vi "Init and Generation Duration.vi"(8 "error in":errorcluster) -> (0 "Generated Error":errorcluster, 2 "Generation Duration [ms]":dbl, 3 "Init Duration [ms]":dbl)   [LabVIEW 2021]
doc: "Measure the duration of <b>Init Error Handler</b> function with 1000 error codes in XML as an input. The resulting duration is returned at <b>Init Duration [ms]</b> output. \nThe time of <b>Generate Error</b> function with no input to format is also measured and returned at <b>Generation Duration [ms]</b> output."
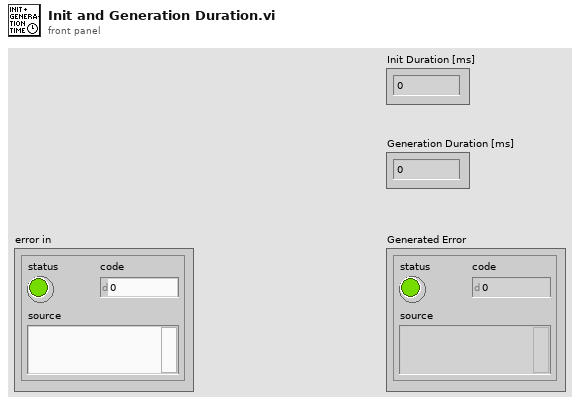
[diagram p1: front panel]
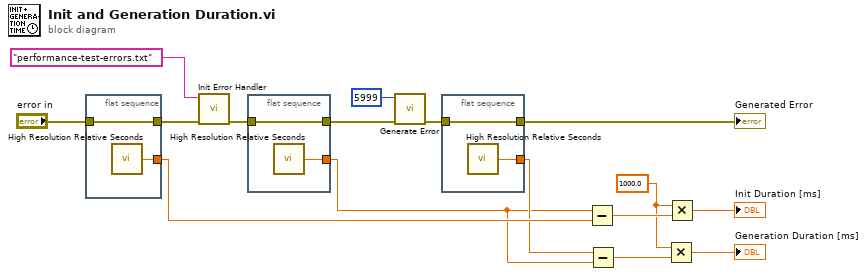
[diagram p0: block diagram]
diagram:
  w6 = 1000.0 ("x")
  n1 = flat-sequence {
    tunnel: [w18] -> w15
    tunnel: "error in" -> [w18]
    tunnel: [w17] -> w12
    frame #0 {
      n2 = call <vilib>:"High Resolution Relative Seconds.vi"() -> ("relative seconds"=w17:dbl)
    }
  }
  n3 = call "Init Error Handler.vi"("error in"=w15, "File Prefix Name (Optional)"="performance-test-errors.txt" ("File Name (Optional)")) -> ("error out"=w13:errorcluster)  [unwired: 9 in]
  n4 = flat-sequence {
    tunnel: [w20] -> w2
    tunnel: w13 -> [w20]
    tunnel: [w19] -> w7
    frame #0 {
      n5 = call <vilib>:"High Resolution Relative Seconds.vi"() -> ("relative seconds"=w19:dbl)
    }
  }
  n6 = call "Generate Error.vi"("error in"=w2, "Error Code"=5999) -> ("Generated Error"=w1:errorcluster)  [unwired: 9 in]
  n7 = flat-sequence {
    tunnel: [w22] -> w10
    tunnel: w1 -> [w22]
    tunnel: [w21] -> w8
    frame #0 {
      n8 = call <vilib>:"High Resolution Relative Seconds.vi"() -> ("relative seconds"=w21:dbl)
    }
  }
  n9 = Subtract(x=w7, y=w12) -> (x-y=w9:dbl)
  n10 = Subtract(x=w8, y=w7) -> (x-y=w5:dbl)
  n11 = Multiply(x=w6, y=w5) -> (x*y=→"Generation Duration [ms]":dbl)
  n12 = Multiply(x=w6, y=w9) -> (x*y=→"Init Duration [ms]":dbl)
  "Generated Error" <- w10
